vi "UPS监控.vi"() -> ()   [LabVIEW 2016, in "环境动力监测库.lvlib" / "UPS库.lvlib"]
uses:
  <vilib>/Utility/miscctls.llb/LVPointTypeDef.ctl
panel:
  in  "变更UPS型号":bool
  out "布尔":bool
  # "UPS监测"
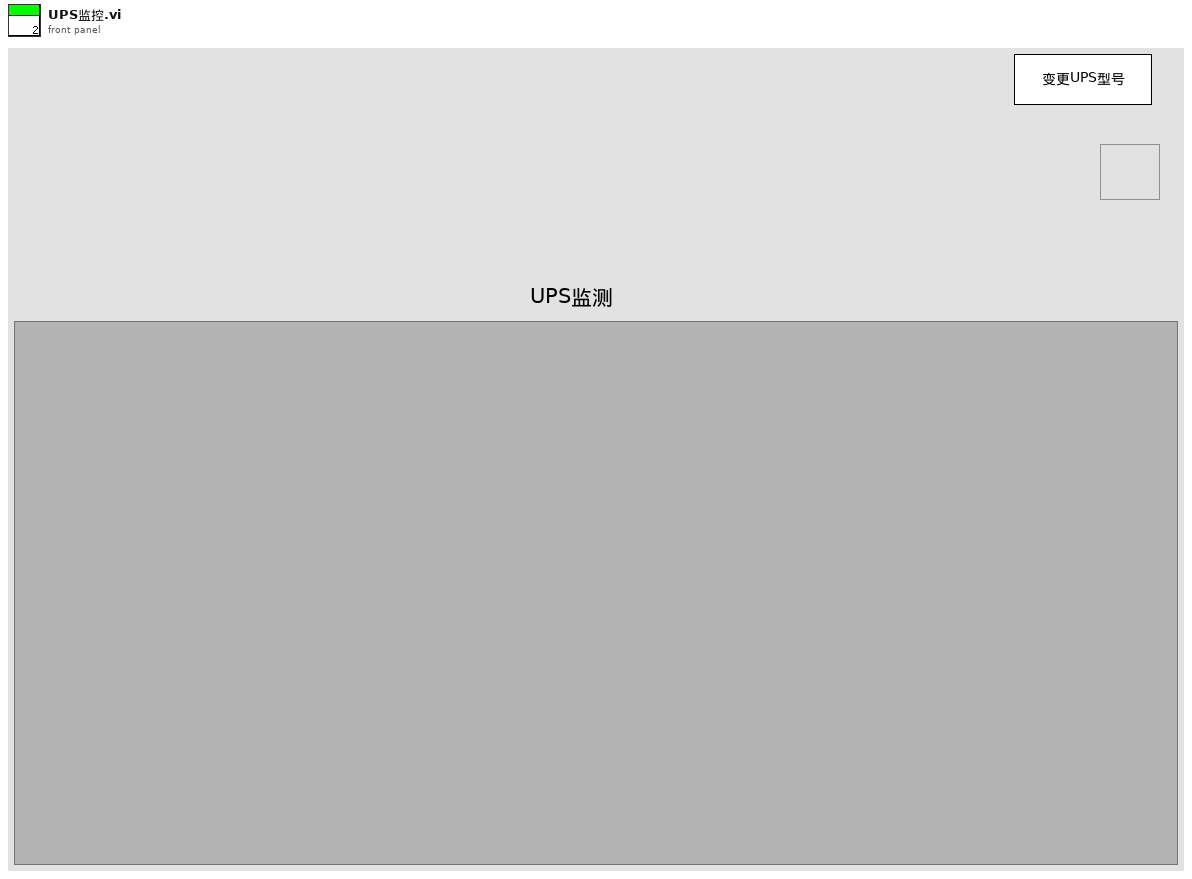
[diagram p1: front panel]
types:
  T1 = enum16{"报警状态监测", "报警确认", "仪器断电", "工控机关机", "取消告警", "结束"}
  T2 = typedef "LVPointTypeDef.ctl" = cluster{"Horizontal":i16, "Vertical":i16}
  T3 = cluster{"VISA resource name":refnum<visa-resource-name>, "Serial Config":cluster{"baud rate (9600)":u32, "stop bits (10: 1 bit)":u16, "parity (0:none)":enum16{"None", "Odd", "Even", "Mark", "Space"}, "data bits (8)":u16, "timeout (10sec)":u32}, "型号选择":enum16{"山特UPSC1~3", "山特UPSC6~20", "华为UPS2000-G-(1-3KVA)"}, "HW-UPS-2000 MB session":refnum<class "MB_Master.lvclass">, "连接方式":enum16{"串口", "TCP"}, "IP":string, "Port":string, "低电量报警阈值":u16, "功能启用":bool}
  T4 = enum16{"山特UPSC1~3", "山特UPSC6~20", "华为UPS2000-G-(1-3KVA)"}
  T5 = enum32{"Bad", "Idle", "Run top level", "Running"}
  T6 = cluster{"输入电压R":dbl, "输入电压S":dbl, "输入电压T":dbl, "输入频率":dbl, "输出电压R":dbl, "输出电压S":dbl, "输出电压T":dbl, "输出频率":dbl, "输出电流R":dbl, "输出电流S":dbl, "输出电流T":dbl, "Positive电池电压":dbl, "Negative电池电压":dbl, "温度":dbl, "电池剩余备用时间":dbl, "电池容量百分比":dbl, "系统模式":dbl, "电池测试状态":dbl, "故障代码":string, "告警":string}
  T7 = cluster{"电池电压V":dbl, "电池状态":u16, "电池剩余容量%":u16, "电池后备时间s":u32, "电池节数":u16, "电池容量AH":u16, "UPS机型KVA":u16}
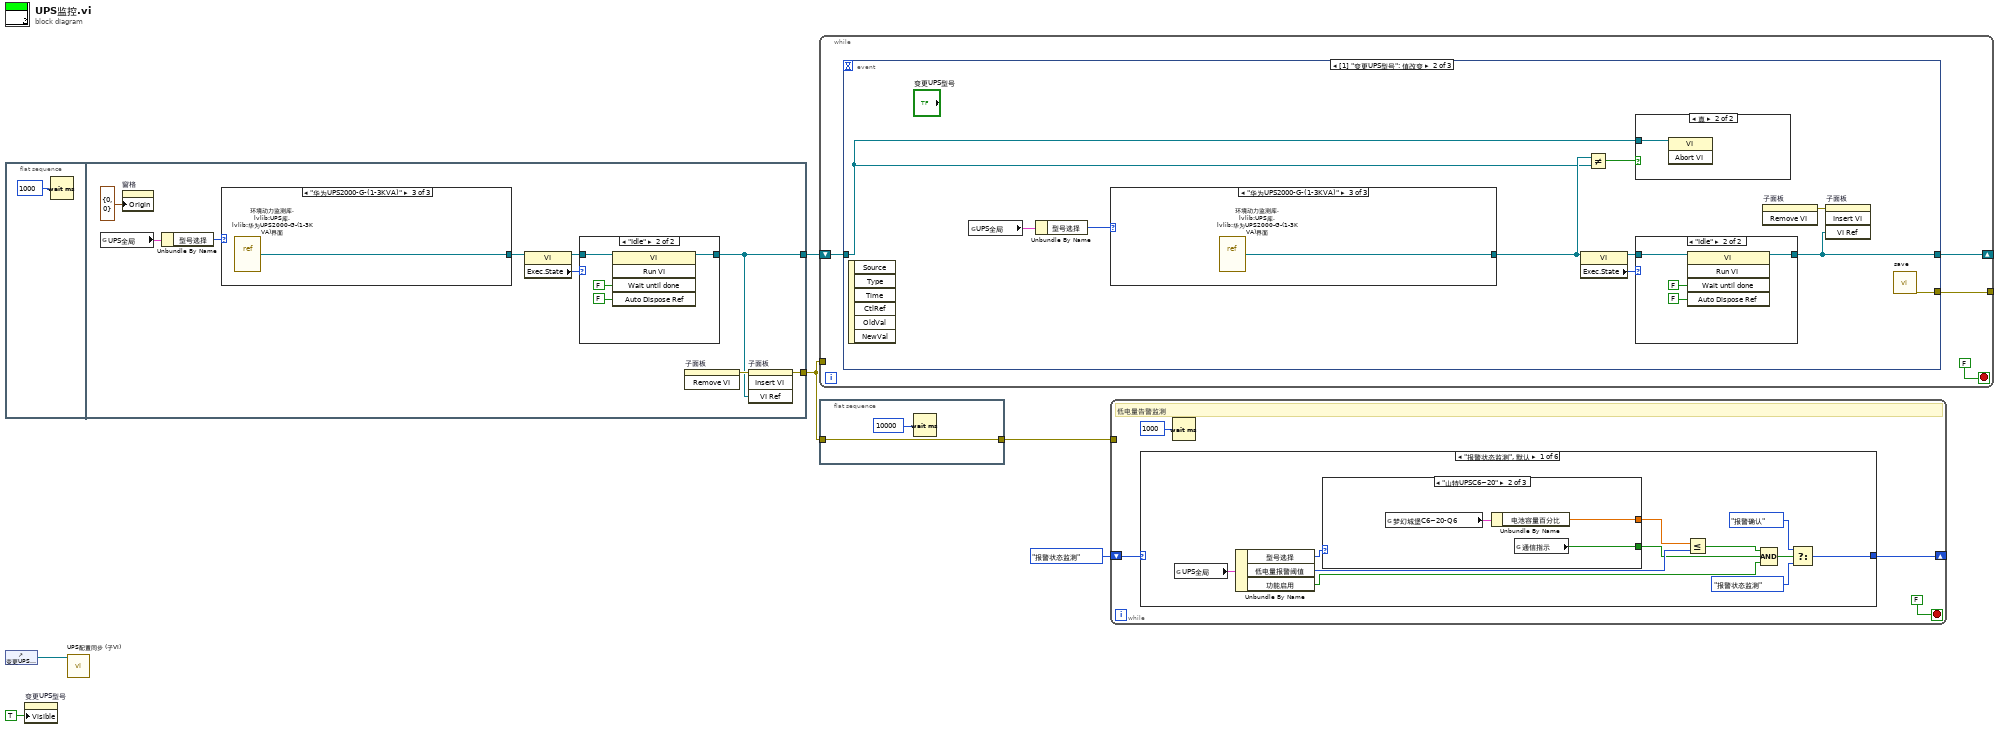
[diagram p0: block diagram]
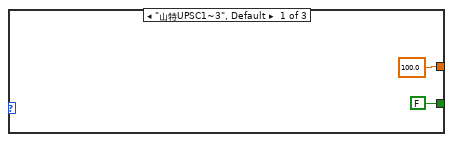
[diagram p2: hidden frame]
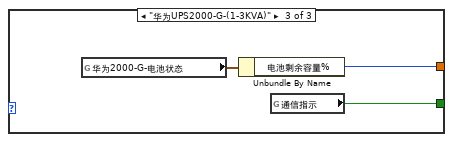
[diagram p3: hidden frame]
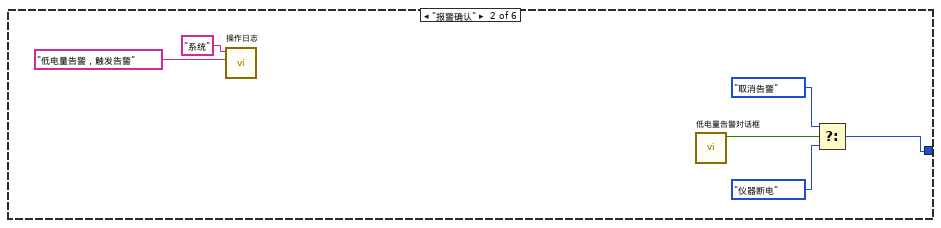
[diagram p4: hidden frame]
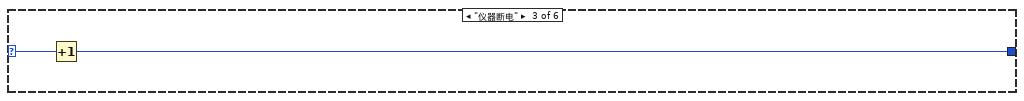
[diagram p5: hidden frame]
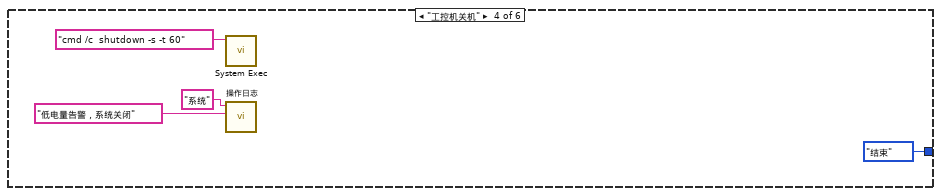
[diagram p6: hidden frame]
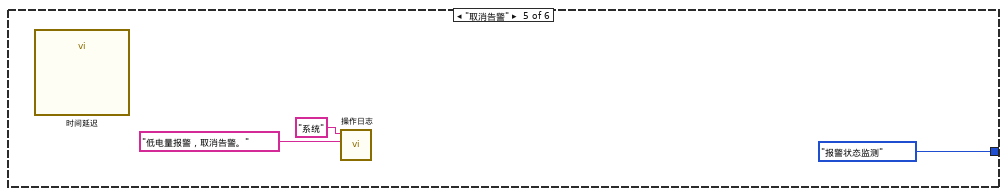
[diagram p7: hidden frame]
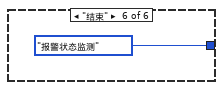
[diagram p8: hidden frame]
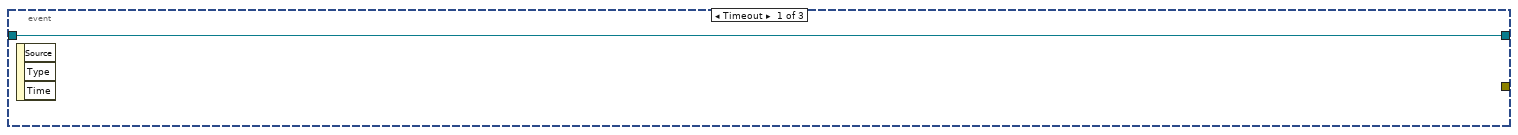
[diagram p9: hidden frame]
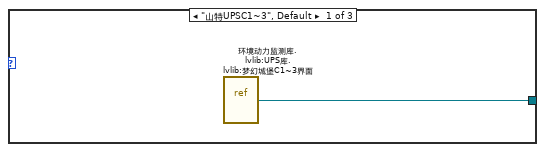
[diagram p11: hidden frame]
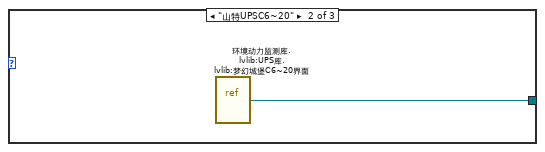
[diagram p12: hidden frame]
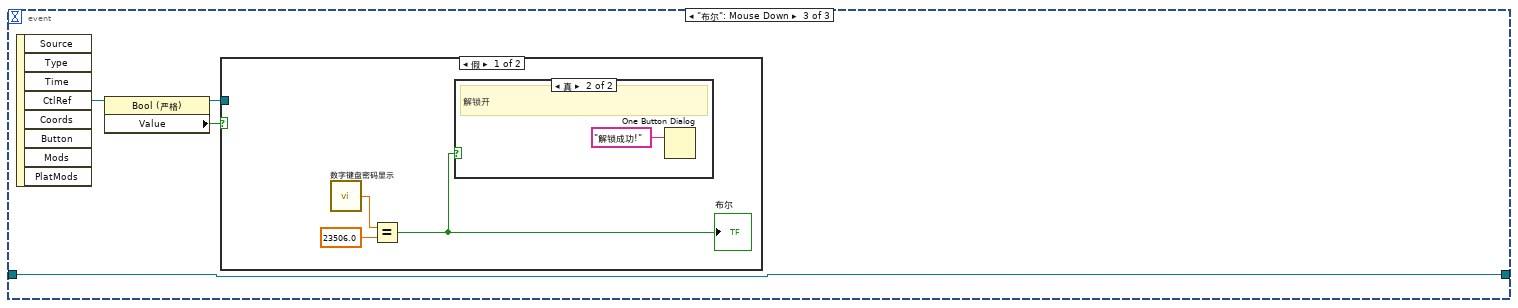
[diagram p14: hidden frame]
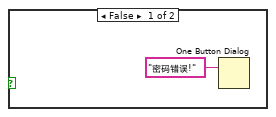
[diagram p15: hidden frame]
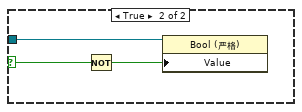
[diagram p16: hidden frame]
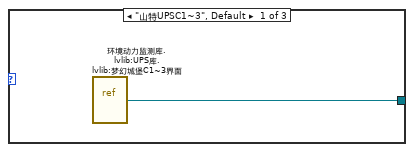
[diagram p17: hidden frame]
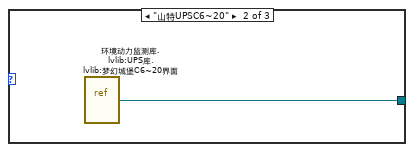
[diagram p18: hidden frame]
diagram:
  n1 = flat-sequence {
    tunnel: [w12] -> w2
    tunnel: [w11] -> w6
    frame #0 {
      n2 = Wait (ms)(milliseconds to wait=u32 1000 ("等待时间（毫秒）")) -> ()  [unwired: 1 out]
    }
    frame #1 {
      n3 = global read "断电保存全局变量.vi" "UPS全局"() -> (w9:T3)
      n4 = property on="窗格" class="Pane"("Origin"=T2 {"Horizontal"=0, "Vertical"=0} ("原点")) -> ()  [unwired: 2 in, 2 out]
      n5 = Unbundle By Name(w9) -> ("型号选择"=w8:T4)
      n6 = case shown="\"华为UPS2000-G-(1-3KVA)\"" w8 {
        tunnel: [w17 w18 w19] -> w14
        frame "山特UPSC1~3", Default {
          n7 = vi-ref "环境动力监测库.lvlib:UPS库.lvlib:梦幻城堡C1~3界面.vi"() -> (w17:refnum<vi>)
        }
        frame "山特UPSC6~20" {
          n8 = vi-ref "环境动力监测库.lvlib:UPS库.lvlib:梦幻城堡C6~20界面.vi"() -> (w18:refnum<vi>)
        }
        frame "华为UPS2000-G-(1-3KVA)" {
          n9 = vi-ref "环境动力监测库.lvlib:UPS库.lvlib:华为UPS2000-G-(1-3KVA)界面.vi"() -> (w19:refnum<vi>)
        }
      }
      n10 = property class="VI"(reference=w14) -> (reference out=w15:refnum<vi>, "Exec.State"=w16:T5)  [unwired: 1 in, 1 out]
      n11 = case shown="\"Idle\"" w16 {
        tunnel: w15 -> [w20 w22]
        tunnel: [w20 w21] -> w11
        frame "Bad", Default {
        }
        frame "Idle" {
          n12 = invoke class="VI" method="Run VI"(reference=w22, "Wait until done"=FALSE ("结束前等待"), "Auto Dispose Ref"=FALSE ("自动销毁引用")) -> (reference out=w21:refnum<vi>)  [unwired: 2 in, 4 out]
        }
      }
      n13 = invoke on="子面板" class="SubPnl" method="Remove VI"() -> (error out=w13:errorcluster)  [unwired: 3 in, 2 out]
      n14 = invoke on="子面板" class="SubPnl" method="Insert VI"(error in=w13, "VI Ref"=w11) -> (error out=w12:errorcluster)  [unwired: 2 in, 3 out]
    }
  }
  n15 = control-ref of="变更UPS型号"() -> (w5:refnum<vi>)
  n16 = property on="变更UPS型号" class="Bool (严格)"("Visible"=TRUE ("可见")) -> ()  [unwired: 2 in, 2 out]
  n17 = call "UPS配置同步 (子VI).vi"("Boolean输入"=w5) -> ()  [unwired: 11 in]
  n18 = while {
    tunnel: w2 -> [_]
    tunnel: [w28] -> _
    shift-right: [w25] -> _
    shift-left: w6 -> [w27]
    stop <- FALSE stop-if-true
    n19 = event shown="[1] \"变更UPS型号\": 值改变" {
      selector: _ -> [_ _ _]
      dyn-events: _ -> [_ _ _]
      timeout: _ -> [_ _ _]
      tunnel: [_ w32 _] -> w28
      tunnel: w27 -> [w29 w33 w49]
      tunnel: [w29 w39 w49] -> w25
      event Timeout {
        n20 = event-data() -> ()  [unwired: 1 in, 3 out]
      }
      event "变更UPS型号": Value Change {
        n21 = event-data() -> ()  [unwired: 1 in, 6 out]
        n22 = global read "断电保存全局变量.vi" "UPS全局"() -> (w31:T3)
        n23 = Unbundle By Name(w31) -> ("型号选择"=w30:T4)
        n24 = case shown="\"华为UPS2000-G-(1-3KVA)\"" w30 {
          tunnel: [w41 w42 w43] -> w35
          frame "山特UPSC1~3", Default {
            n25 = vi-ref "环境动力监测库.lvlib:UPS库.lvlib:梦幻城堡C1~3界面.vi"() -> (w41:refnum<vi>)
          }
          frame "山特UPSC6~20" {
            n26 = vi-ref "环境动力监测库.lvlib:UPS库.lvlib:梦幻城堡C6~20界面.vi"() -> (w42:refnum<vi>)
          }
          frame "华为UPS2000-G-(1-3KVA)" {
            n27 = vi-ref "环境动力监测库.lvlib:UPS库.lvlib:华为UPS2000-G-(1-3KVA)界面.vi"() -> (w43:refnum<vi>)
          }
        }
        n28 = property class="VI"(reference=w35) -> (reference out=w37:refnum<vi>, "Exec.State"=w38:T5)  [unwired: 1 in, 1 out]
        n29 = Not Equal?(x=w35, y=w33) -> (x != y?=w34:bool)
        n30 = case shown="真" w34 {
          tunnel: w33 -> [_ w40]
          frame False {
          }
          frame True {
            n31 = invoke class="VI" method="Abort VI"(reference=w40) -> ()  [unwired: 2 in, 3 out]
          }
        }
        n32 = case shown="\"Idle\"" w38 {
          tunnel: w37 -> [w44 w46]
          tunnel: [w44 w45] -> w39
          frame "Bad", Default {
          }
          frame "Idle" {
            n33 = invoke class="VI" method="Run VI"(reference=w46, "Wait until done"=FALSE ("结束前等待"), "Auto Dispose Ref"=FALSE ("自动销毁引用")) -> (reference out=w45:refnum<vi>)  [unwired: 2 in, 4 out]
          }
        }
        n34 = invoke on="子面板" class="SubPnl" method="Remove VI"() -> (error out=w36:errorcluster)  [unwired: 3 in, 2 out]
        n35 = invoke on="子面板" class="SubPnl" method="Insert VI"(error in=w36, "VI Ref"=w39) -> ()  [unwired: 2 in, 4 out]
        n36 = call "save.vi"() -> ("error out"=w32:errorcluster)  [unwired: 11 in]
      }
      event "布尔": Mouse Down {
        n37 = event-data() -> ("CtlRef"=w52:refnum<vi>)  [unwired: 1 in, 7 out]
        n38 = property class="Bool (严格)"(reference=w52) -> (reference out=w50:refnum<vi>, "Value"=w51:bool)  [unwired: 1 in, 1 out]
        n39 = case shown="假" w51 {
          selector: w51 -> [_ w59]
          tunnel: w50 -> [_ w60]
          frame False {
            n40 = call "数字键盘密码显示.vi"() -> ("NewNumber"=w55:sgl)  [unwired: 1 in]
            n41 = Equal?(x=w55, y=sgl 23506.0) -> (x = y?=w53:bool)
            "布尔" <- w53
            n42 = case shown="真" w53 {
              frame False {
                n43 = One Button Dialog(message="密码错误!" ("消息")) -> ()  [unwired: 1 in, 1 out]
              }
              frame True {
                # "解锁开"
                n44 = One Button Dialog(message="解锁成功!" ("消息")) -> ()  [unwired: 1 in, 1 out]
              }
            }
          }
          frame True {
            n45 = Not(x=w59) -> (.not. x?=w58:bool)
            n46 = property class="Bool (严格)"(reference=w60, "Value"=w58) -> ()  [unwired: 1 in, 2 out]
          }
        }
      }
    }
  }
  n47 = flat-sequence {
    tunnel: w2 -> [w62]
    tunnel: [w62] -> w1
    frame #0 {
      n48 = Wait (ms)(milliseconds to wait=u32 10000 ("等待时间（毫秒）")) -> ()  [unwired: 1 out]
    }
  }
  n49 = while {
    shift-right: [w66] -> _
    shift-left: T1."报警状态监测" ("枚举") -> [w65]
    tunnel: w1 -> [_]
    stop <- FALSE stop-if-true
    # "低电量告警监测"
    n50 = case shown="\"报警状态监测\", 默认" w65 {
      selector: w65 -> [_ _ w93 _ _ _]
      tunnel: [w70 w88 w92 T1."结束" ("枚举") T1."报警状态监测" ("枚举") T1."报警状态监测" ("枚举")] -> w66
      frame "报警状态监测", Default {
        n51 = global read "断电保存全局变量.vi" "UPS全局"() -> (w77:T3)
        n52 = Unbundle By Name(w77) -> ("型号选择"=w76:T4, "低电量报警阈值"=w74:u16, "功能启用"=w67:bool)
        n53 = case shown="\"山特UPSC6~20\"" w76 {
          tunnel: [100.0 ("电池容量百分比") w81 w84] -> w75
          tunnel: [FALSE ("通信指示") w80 w83] -> w68
          frame "山特UPSC1~3", Default {
          }
          frame "山特UPSC6~20" {
            n54 = global read "UPS内部交互全局.vi" "梦幻城堡C6~20-Q6"() -> (w82:T6)
            n55 = Unbundle By Name(w82) -> ("电池容量百分比"=w81:dbl)
            n56 = global read "UPS内部交互全局.vi" "通信指示"() -> (w80:bool)
          }
          frame "华为UPS2000-G-(1-3KVA)" {
            n57 = global read "UPS内部交互全局.vi" "华为2000-G-电池状态"() -> (w85:T7)
            n58 = Unbundle By Name(w85) -> ("电池剩余容量%"=w84:u16)
            n59 = global read "UPS内部交互全局.vi" "通信指示"() -> (w83:bool)
          }
        }
        n60 = Less Or Equal?(x=w75, y=w74) -> (x <= y?=w73:bool)
        n61 = Compound Arithmetic op=AND ("复合运算")(w73, w68, w67) -> (w69:bool)
        n62 = Select(t=T1."报警确认" ("枚举"), s=w69, f=T1."报警状态监测" ("枚举")) -> (s? t:f=w70:T1)
      }
      frame "报警确认" {
        n63 = call "操作日志.vi"("日志信息"="低电量告警，触发告警", "设备"="系统") -> ()  [unwired: 9 in, 1 out]
        n64 = call "低电量告警对话框.vi"() -> ("T button?"=w91:bool)  [unwired: 11 in]
        n65 = Select(t=T1."取消告警" ("枚举"), s=w91, f=T1."仪器断电" ("枚举")) -> (s? t:f=w88:T1)
      }
      frame "仪器断电" {
        n66 = Increment(x=w93) -> (x+1=w92:T1)
      }
      frame "工控机关机" {
        n67 = call <vilib>:"System Exec.vi"("command line"="cmd /c  shutdown -s -t 60") -> ()  [unwired: 7 in, 4 out]
        n68 = call "操作日志.vi"("日志信息"="低电量告警，系统关闭", "设备"="系统") -> ()  [unwired: 9 in, 1 out]
      }
      frame "取消告警" {
        n69 = call "时间延迟"() -> ()  [unwired: 11 in, 1 out]
        n70 = call "操作日志.vi"("日志信息"="低电量报警，取消告警。", "设备"="系统") -> ()  [unwired: 9 in, 1 out]
      }
      frame "结束" {
      }
    }
    n71 = Wait (ms)(milliseconds to wait=u32 1000 ("等待时间（毫秒）")) -> ()  [unwired: 1 out]
  }
